vi "HUI v0.2.vi"() -> ()   [LabVIEW 2016]
uses:
  <vilib>/measure/NI_MABase.lvlib
panel:
  out "hui":dbl[](array[numeric])
  in  "wait":u32
  out "Point free":u32
  out "Point processed":u32
  in  "Quant":i32=100
  in  "stop":bool
  out "DAC FREQ/CH, Hz":dbl
  out "String":string
  in  "STOP_RUN":bool
  in  "FREQ":dbl(knob)=100.0 scale=0.0..100000.0
  in  "SIZE":dbl(knob)=1.0 scale=0.0..5.0
  # "CHANNEL A"
  # "CHANNEL B"
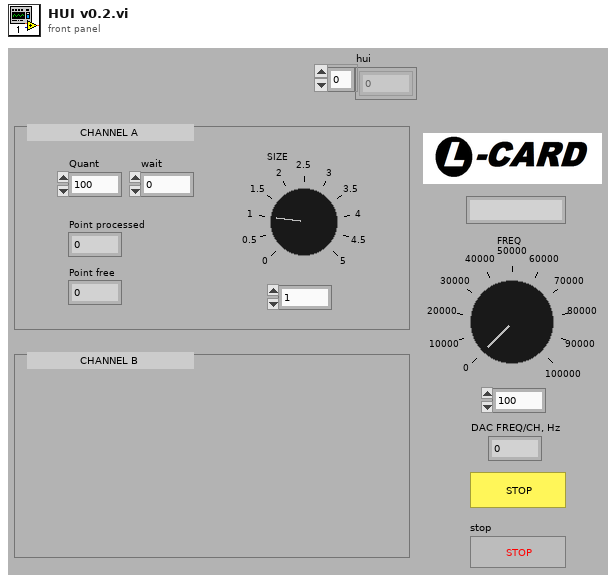
[diagram p1: front panel]
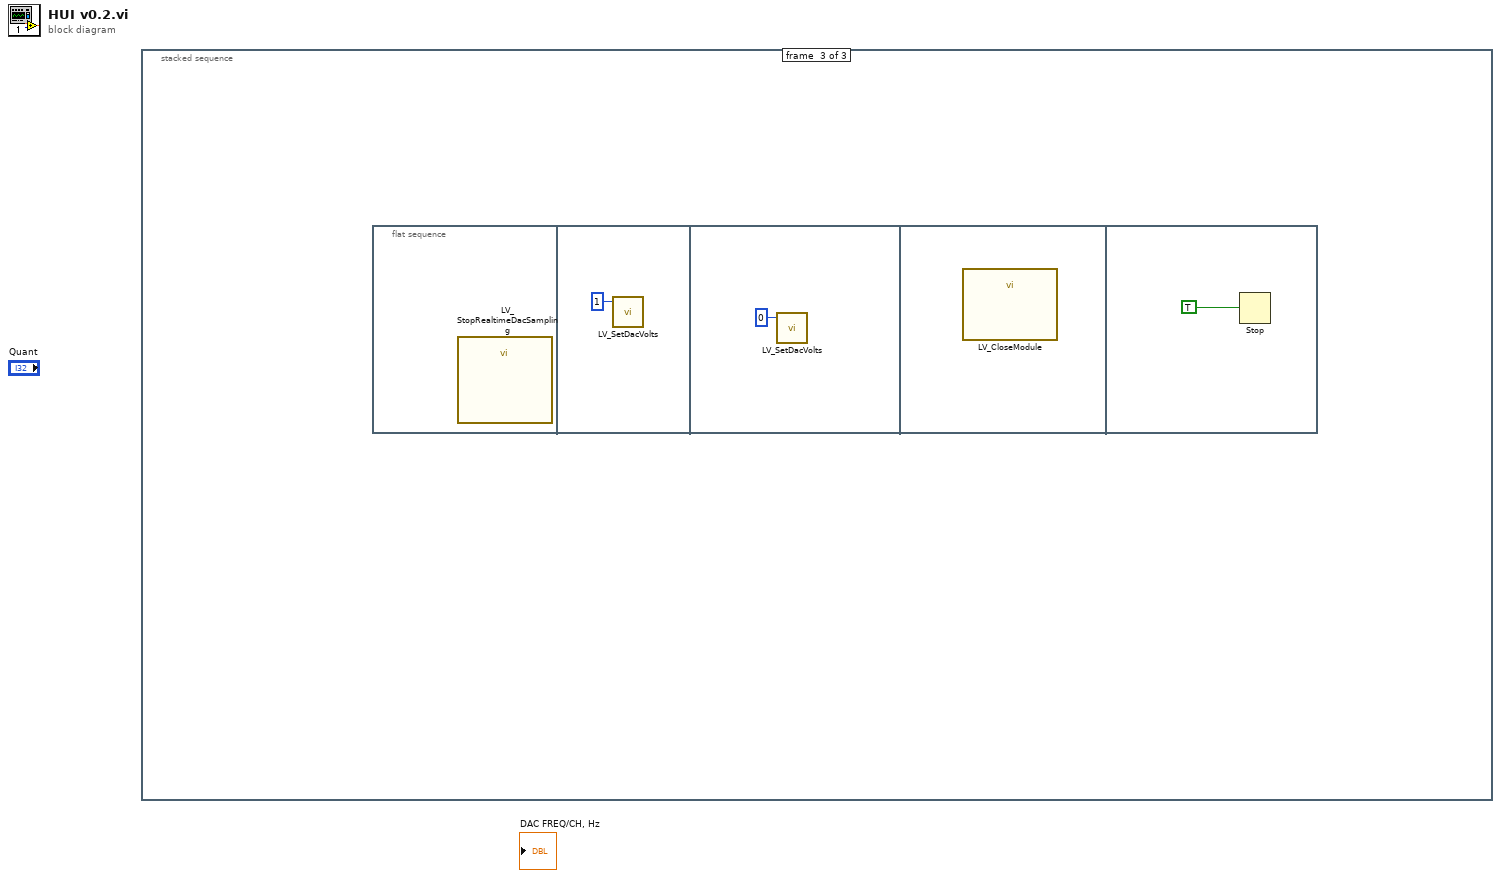
[diagram p0: block diagram]
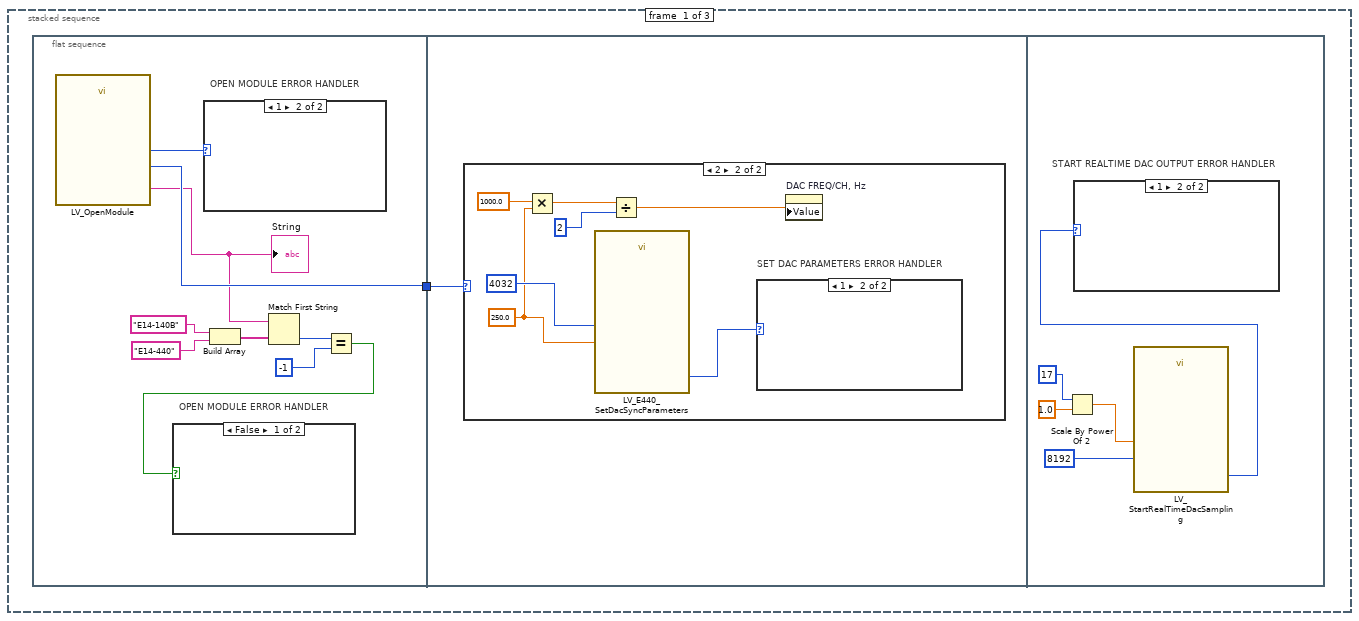
[diagram p2: hidden frame]
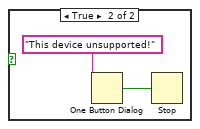
[diagram p3: hidden frame]
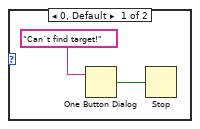
[diagram p4: hidden frame]
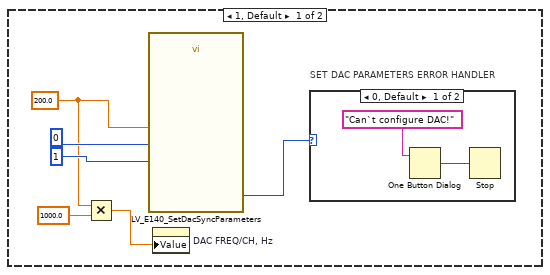
[diagram p5: hidden frame]
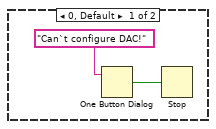
[diagram p7: hidden frame]
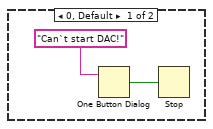
[diagram p8: hidden frame]
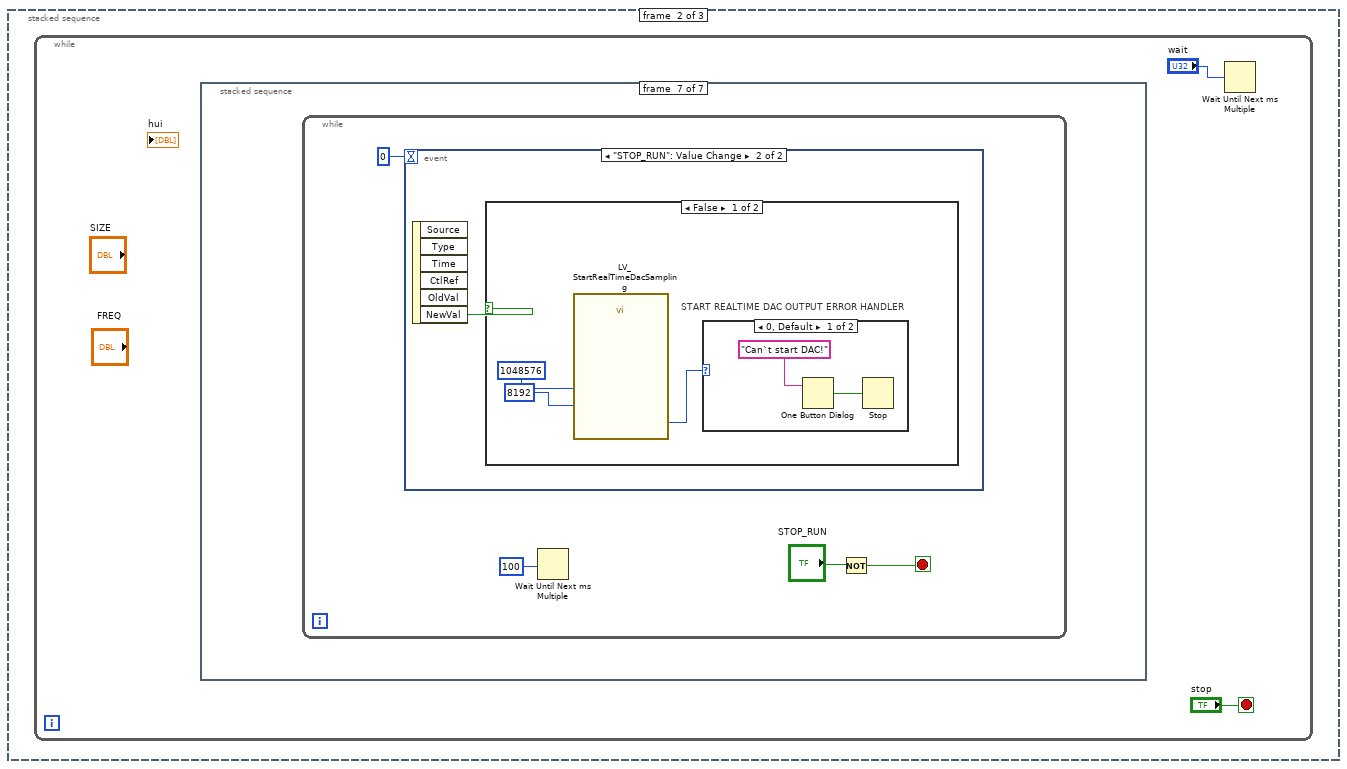
[diagram p9: hidden frame]
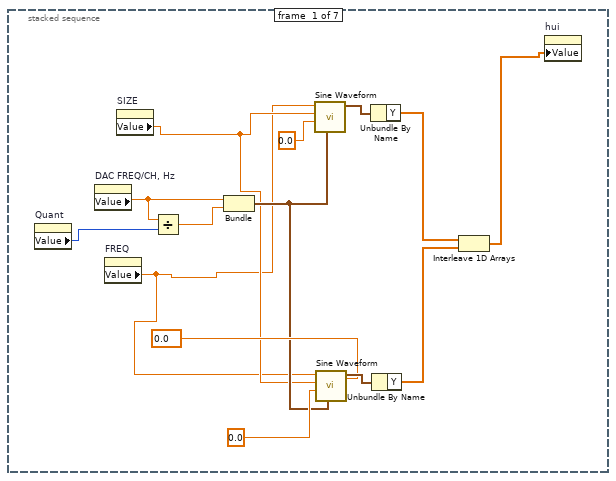
[diagram p10: hidden frame]
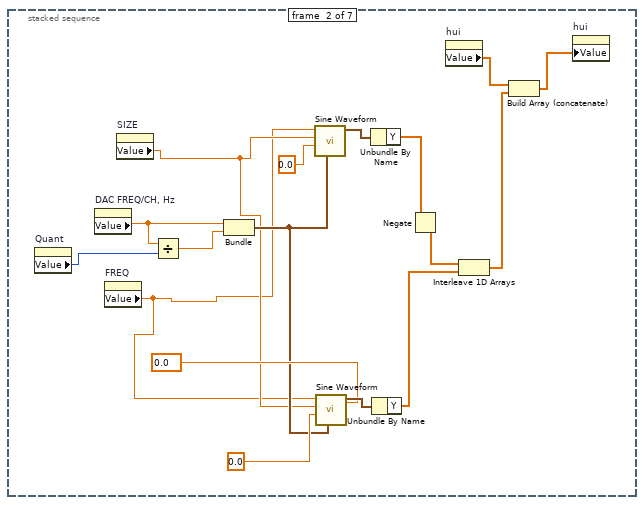
[diagram p11: hidden frame]
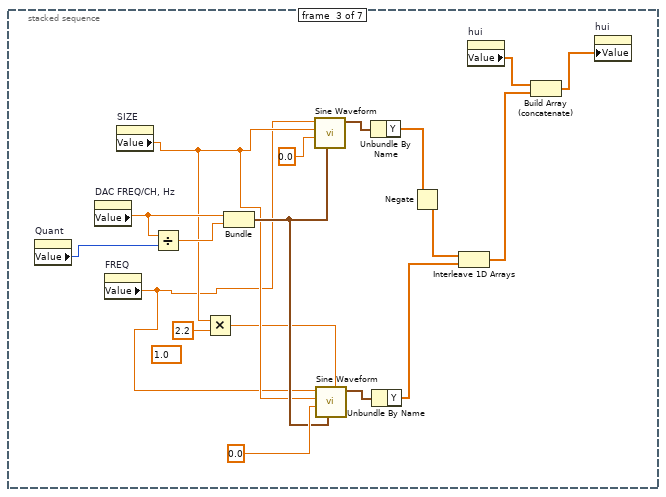
[diagram p12: hidden frame]
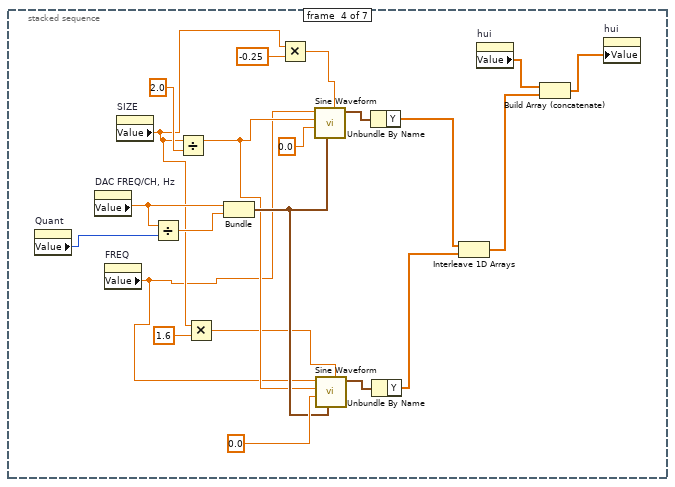
[diagram p13: hidden frame]
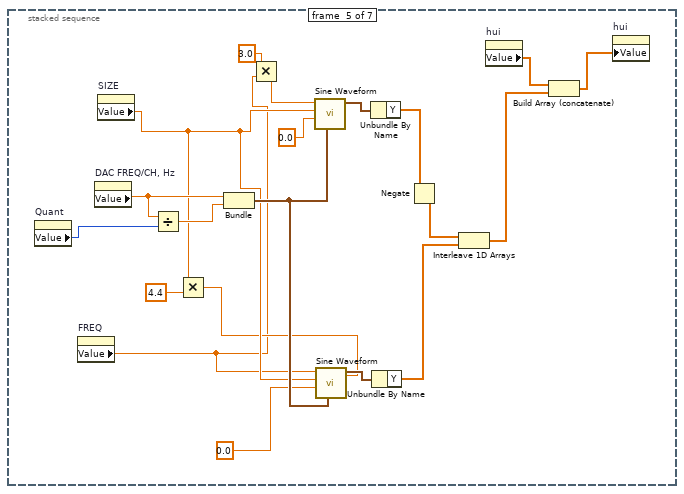
[diagram p14: hidden frame]
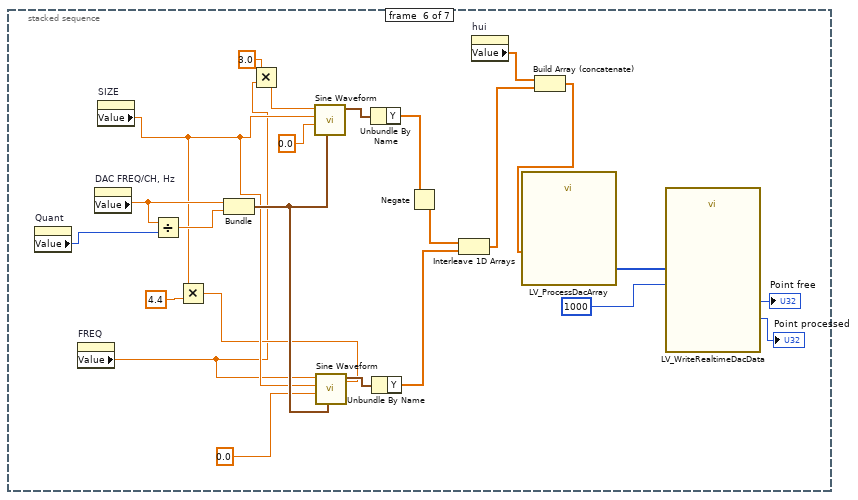
[diagram p15: hidden frame]
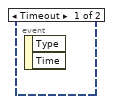
[diagram p16: hidden frame]
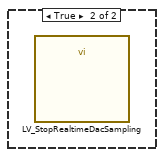
[diagram p18: hidden frame]
diagram:
  n1 = stacked-sequence {
    frame #0 {
      n2 = flat-sequence {
        tunnel: [w3] -> w1
        tunnel: w1 -> [w15]
        frame #0 {
          n3 = call <instrlib>:"LV_OpenModule.vi"() -> ("Module Name"=w2:string, "Module id"=w3:u8, "Error"=w4:u8)
          "String" <- w2
          n4 = case "OPEN MODULE ERROR HANDLER" shown="1" w4 {
            frame 0, Default {
              n5 = One Button Dialog(message="Can`t find target!") -> (true=w13:bool)  [unwired: 1 in]
              n6 = Stop(stop? (T)=w13) -> ()
            }
            frame 1 {
            }
          }
          n7 = Build Array("E14-140B", "E14-440") -> (w8:string[])
          n8 = Match First String(2:w8, 3:w2) -> (0:w7:i32)  [unwired: 1 out]
          n9 = Equal?(x=w7, y=-1) -> (x = y?=w5:bool)
          n10 = case "OPEN MODULE ERROR HANDLER" shown="False" w5 {
            frame False {
            }
            frame True {
              n11 = One Button Dialog(message="This device unsupported!") -> (true=w12:bool)  [unwired: 1 in]
              n12 = Stop(stop? (T)=w12) -> ()
            }
          }
        }
        frame #1 {
          n13 = case shown="2" w15 {
            frame 1, Default {
              w16 = 200.0
              n14 = Multiply(x=w16, y=1000.0) -> (x*y=w18:dbl)
              n15 = call <instrlib>:"LV_E140_SetDacSyncParameters.vi"("Zero on stop"=1, "Sync with ADC"=0, "Rate"=w16) -> ("Error"=w19:u32)  [unwired: 1 out]
              n16 = property on="DAC FREQ/CH, Hz" class="DigNum (strict)"("Value"=w18) -> ()  [unwired: 2 in, 2 out]
              n17 = case "SET DAC PARAMETERS ERROR HANDLER" shown="0, Default" w19 {
                frame 0, Default {
                  n18 = One Button Dialog(message="Can`t configure DAC!") -> (true=w22:bool)  [unwired: 1 in]
                  n19 = Stop(stop? (T)=w22) -> ()
                }
                frame 1 {
                }
              }
            }
            frame 2 {
              w25 = 250.0
              n20 = Multiply(x=1000.0, y=w25) -> (x*y=w26:dbl)
              n21 = call <instrlib>:"LV_E440_SetDacSyncParameters.vi"("Fifo length"=4032, "Rate"=w25) -> ("Error"=w27:u32)  [unwired: 1 out]
              n22 = Divide(x=w26, y=2) -> (x/y=w30:dbl)
              n23 = case "SET DAC PARAMETERS ERROR HANDLER" shown="1" w27 {
                frame 0, Default {
                  n24 = One Button Dialog(message="Can`t configure DAC!") -> (true=w31:bool)  [unwired: 1 in]
                  n25 = Stop(stop? (T)=w31) -> ()
                }
                frame 1 {
                }
              }
              n26 = property on="DAC FREQ/CH, Hz" class="DigNum (strict)"("Value"=w30) -> ()  [unwired: 2 in, 2 out]
            }
          }
        }
        frame #2 {
          n27 = Scale By Power Of 2(n=i16 17, x=1.0) -> (x*2^n=w33:dbl)
          n28 = call <instrlib>:"LV_StartRealTimeDacSampling.vi"("Packet size"=8192, "Buffer Size"=w33) -> ("Error"=w36:u8)
          n29 = case "START REALTIME DAC OUTPUT ERROR HANDLER" shown="1" w36 {
            frame 0, Default {
              n30 = One Button Dialog(message="Can`t start DAC!") -> (true=w38:bool)  [unwired: 1 in]
              n31 = Stop(stop? (T)=w38) -> ()
            }
            frame 1 {
            }
          }
        }
      }
    }
    frame #1 {
      n32 = while {
        stop <- "stop" stop-if-true
        n33 = stacked-sequence {
          frame #0 {
            w52 = 0.0 items=["-5V"=-5.0, "-2V"=-2.0, "-1V"=-1.0, "0V"=0.0, "1V"=1.0, "2V"=2.0, "5V"=5.0] ("DC OFFSET")
            n34 = property on="Quant" class="DigNum (strict)"() -> ("Value"=w46:i32)  [unwired: 2 in, 2 out]
            n35 = property on="DAC FREQ/CH, Hz" class="DigNum (strict)"() -> ("Value"=w49:dbl)  [unwired: 2 in, 2 out]
            n36 = property on="FREQ" class="Knob (strict)"() -> ("Value"=w43:dbl)  [unwired: 2 in, 2 out]
            n37 = property on="SIZE" class="Knob (strict)"() -> ("Value"=w44:dbl)  [unwired: 2 in, 2 out]
            n38 = Divide(x=w49, y=w46) -> (x/y=w48:dbl)
            n39 = Bundle("Value"=w49, w48) -> (w45:cluster{"Value":dbl, dbl})  [unwired: 1 in]
            n40 = call <vilib>:"Sine Waveform.vi"("sampling info"=w45, "phase"=sgl 0.0, "amplitude"=w44, "frequency"=w43) -> ("signal out"=w55:waveform(dbl))  [unwired: 6 in, 1 out]
            n41 = call <vilib>:"Sine Waveform.vi"("offset"=w52, "sampling info"=w45, "phase"=0.0, "amplitude"=w44, "frequency"=w43) -> ("signal out"=w53:waveform(dbl))  [unwired: 5 in, 1 out]
            n42 = Unbundle By Name(w55) -> ("Y"=w51:dbl[])
            n43 = Unbundle By Name(w53) -> ("Y"=w50:dbl[])
            n44 = Interleave 1D Arrays(w51, w50) -> (w42:dbl[])
            n45 = property on="hui" class="Arr (strict)"("Value"=w42) -> ()  [unwired: 2 in, 2 out]
          }
          frame #1 {
            w69 = 0.0 items=["-5V"=-5.0, "-2V"=-2.0, "-1V"=-1.0, "0V"=0.0, "1V"=1.0, "2V"=2.0, "5V"=5.0] ("DC OFFSET")
            n46 = property on="Quant" class="DigNum (strict)"() -> ("Value"=w63:i32)  [unwired: 2 in, 2 out]
            n47 = property on="DAC FREQ/CH, Hz" class="DigNum (strict)"() -> ("Value"=w66:dbl)  [unwired: 2 in, 2 out]
            n48 = property on="FREQ" class="Knob (strict)"() -> ("Value"=w60:dbl)  [unwired: 2 in, 2 out]
            n49 = property on="SIZE" class="Knob (strict)"() -> ("Value"=w61:dbl)  [unwired: 2 in, 2 out]
            n50 = Divide(x=w66, y=w63) -> (x/y=w65:dbl)
            n51 = Bundle("Value"=w66, w65) -> (w62:cluster{"Value":dbl, dbl})  [unwired: 1 in]
            n52 = call <vilib>:"Sine Waveform.vi"("sampling info"=w62, "phase"=sgl 0.0, "amplitude"=w61, "frequency"=w60) -> ("signal out"=w72:waveform(dbl))  [unwired: 6 in, 1 out]
            n53 = call <vilib>:"Sine Waveform.vi"("offset"=w69, "sampling info"=w62, "phase"=0.0, "amplitude"=w61, "frequency"=w60) -> ("signal out"=w70:waveform(dbl))  [unwired: 5 in, 1 out]
            n54 = Unbundle By Name(w72) -> ("Y"=w68:dbl[])
            n55 = Unbundle By Name(w70) -> ("Y"=w67:dbl[])
            n56 = Negate(x=w68) -> (-x=w58:dbl[])
            n57 = property on="hui" class="Arr (strict)"() -> ("Value"=w57:dbl[])  [unwired: 2 in, 2 out]
            n58 = Interleave 1D Arrays(w58, w67) -> (w59:dbl[])
            n59 = Build Array (concatenate)(w57, w59) -> (w56:dbl[])
            n60 = property on="hui" class="Arr (strict)"("Value"=w56) -> ()  [unwired: 2 in, 2 out]
          }
          frame #2 {
            (unwired) 1.0 items=["-5V"=-5.0, "-2V"=-2.0, "-1V"=-1.0, "0V"=0.0, "1V"=1.0, "2V"=2.0, "5V"=5.0] ("DC OFFSET")
            n61 = property on="Quant" class="DigNum (strict)"() -> ("Value"=w82:i32)  [unwired: 2 in, 2 out]
            n62 = property on="DAC FREQ/CH, Hz" class="DigNum (strict)"() -> ("Value"=w85:dbl)  [unwired: 2 in, 2 out]
            n63 = property on="FREQ" class="Knob (strict)"() -> ("Value"=w76:dbl)  [unwired: 2 in, 2 out]
            n64 = property on="SIZE" class="Knob (strict)"() -> ("Value"=w78:dbl)  [unwired: 2 in, 2 out]
            n65 = Divide(x=w85, y=w82) -> (x/y=w84:dbl)
            n66 = Multiply(x=w78, y=2.2) -> (x*y=w77:dbl)
            n67 = Bundle("Value"=w85, w84) -> (w81:cluster{"Value":dbl, dbl})  [unwired: 1 in]
            n68 = call <vilib>:"Sine Waveform.vi"("sampling info"=w81, "phase"=sgl 0.0, "amplitude"=w78, "frequency"=w76) -> ("signal out"=w90:waveform(dbl))  [unwired: 6 in, 1 out]
            n69 = call <vilib>:"Sine Waveform.vi"("offset"=w77, "sampling info"=w81, "phase"=0.0, "amplitude"=w78, "frequency"=w76) -> ("signal out"=w88:waveform(dbl))  [unwired: 5 in, 1 out]
            n70 = Unbundle By Name(w90) -> ("Y"=w87:dbl[])
            n71 = Unbundle By Name(w88) -> ("Y"=w86:dbl[])
            n72 = Negate(x=w87) -> (-x=w80:dbl[])
            n73 = Interleave 1D Arrays(w80, w86) -> (w73:dbl[])
            n74 = property on="hui" class="Arr (strict)"() -> ("Value"=w75:dbl[])  [unwired: 2 in, 2 out]
            n75 = Build Array (concatenate)(w75, w73) -> (w74:dbl[])
            n76 = property on="hui" class="Arr (strict)"("Value"=w74) -> ()  [unwired: 2 in, 2 out]
          }
          frame #3 {
            n77 = property on="Quant" class="DigNum (strict)"() -> ("Value"=w103:i32)  [unwired: 2 in, 2 out]
            n78 = property on="DAC FREQ/CH, Hz" class="DigNum (strict)"() -> ("Value"=w106:dbl)  [unwired: 2 in, 2 out]
            n79 = property on="FREQ" class="Knob (strict)"() -> ("Value"=w94:dbl)  [unwired: 2 in, 2 out]
            n80 = property on="SIZE" class="Knob (strict)"() -> ("Value"=w96:dbl)  [unwired: 2 in, 2 out]
            n81 = Divide(x=w106, y=w103) -> (x/y=w105:dbl)
            n82 = Divide(x=w96, y=2.0) -> (x/y=w101:dbl)
            n83 = Multiply(x=w96, y=1.6) -> (x*y=w98:dbl)
            n84 = Bundle("Value"=w106, w105) -> (w102:cluster{"Value":dbl, dbl})  [unwired: 1 in]
            n85 = Multiply(x=w96, y=-0.25) -> (x*y=w95:dbl)
            n86 = call <vilib>:"Sine Waveform.vi"("offset"=w95, "sampling info"=w102, "phase"=sgl 0.0, "amplitude"=w101, "frequency"=w94) -> ("signal out"=w111:waveform(dbl))  [unwired: 5 in, 1 out]
            n87 = call <vilib>:"Sine Waveform.vi"("offset"=w98, "sampling info"=w102, "phase"=0.0, "amplitude"=w101, "frequency"=w94) -> ("signal out"=w109:waveform(dbl))  [unwired: 5 in, 1 out]
            n88 = Unbundle By Name(w111) -> ("Y"=w108:dbl[])
            n89 = Unbundle By Name(w109) -> ("Y"=w107:dbl[])
            n90 = Interleave 1D Arrays(w108, w107) -> (w91:dbl[])
            n91 = property on="hui" class="Arr (strict)"() -> ("Value"=w92:dbl[])  [unwired: 2 in, 2 out]
            n92 = Build Array (concatenate)(w92, w91) -> (w93:dbl[])
            n93 = property on="hui" class="Arr (strict)"("Value"=w93) -> ()  [unwired: 2 in, 2 out]
          }
          frame #4 {
            n94 = property on="Quant" class="DigNum (strict)"() -> ("Value"=w124:i32)  [unwired: 2 in, 2 out]
            n95 = property on="FREQ" class="Knob (strict)"() -> ("Value"=w116:dbl)  [unwired: 2 in, 2 out]
            n96 = property on="DAC FREQ/CH, Hz" class="DigNum (strict)"() -> ("Value"=w126:dbl)  [unwired: 2 in, 2 out]
            n97 = property on="SIZE" class="Knob (strict)"() -> ("Value"=w120:dbl)  [unwired: 2 in, 2 out]
            n98 = Divide(x=w126, y=w124) -> (x/y=w125:dbl)
            n99 = Multiply(x=w120, y=4.4) -> (x*y=w119:dbl)
            n100 = Bundle("Value"=w126, w125) -> (w123:cluster{"Value":dbl, dbl})  [unwired: 1 in]
            n101 = Multiply(x=3.0 ("frequency"), y=w116) -> (x*y=w117:dbl)
            n102 = call <vilib>:"Sine Waveform.vi"("sampling info"=w123, "phase"=sgl 0.0, "amplitude"=w120, "frequency"=w117) -> ("signal out"=w131:waveform(dbl))  [unwired: 6 in, 1 out]
            n103 = call <vilib>:"Sine Waveform.vi"("offset"=w119, "sampling info"=w123, "phase"=0.0, "amplitude"=w120, "frequency"=w116) -> ("signal out"=w129:waveform(dbl))  [unwired: 5 in, 1 out]
            n104 = Unbundle By Name(w131) -> ("Y"=w128:dbl[])
            n105 = Unbundle By Name(w129) -> ("Y"=w127:dbl[])
            n106 = Negate(x=w128) -> (-x=w115:dbl[])
            n107 = Interleave 1D Arrays(w115, w127) -> (w112:dbl[])
            n108 = property on="hui" class="Arr (strict)"() -> ("Value"=w114:dbl[])  [unwired: 2 in, 2 out]
            n109 = Build Array (concatenate)(w114, w112) -> (w113:dbl[])
            n110 = property on="hui" class="Arr (strict)"("Value"=w113) -> ()  [unwired: 2 in, 2 out]
          }
          frame #5 {
            n111 = property on="Quant" class="DigNum (strict)"() -> ("Value"=w146:i32)  [unwired: 2 in, 2 out]
            n112 = property on="FREQ" class="Knob (strict)"() -> ("Value"=w138:dbl)  [unwired: 2 in, 2 out]
            n113 = property on="DAC FREQ/CH, Hz" class="DigNum (strict)"() -> ("Value"=w150:dbl)  [unwired: 2 in, 2 out]
            n114 = property on="SIZE" class="Knob (strict)"() -> ("Value"=w142:dbl)  [unwired: 2 in, 2 out]
            n115 = Divide(x=w150, y=w146) -> (x/y=w149:dbl)
            n116 = Multiply(x=w142, y=4.4) -> (x*y=w141:dbl)
            n117 = Bundle("Value"=w150, w149) -> (w145:cluster{"Value":dbl, dbl})  [unwired: 1 in]
            n118 = Multiply(x=3.0 ("frequency"), y=w138) -> (x*y=w139:dbl)
            n119 = call <vilib>:"Sine Waveform.vi"("sampling info"=w145, "phase"=sgl 0.0, "amplitude"=w142, "frequency"=w139) -> ("signal out"=w155:waveform(dbl))  [unwired: 6 in, 1 out]
            n120 = call <vilib>:"Sine Waveform.vi"("offset"=w141, "sampling info"=w145, "phase"=0.0, "amplitude"=w142, "frequency"=w138) -> ("signal out"=w153:waveform(dbl))  [unwired: 5 in, 1 out]
            n121 = Unbundle By Name(w155) -> ("Y"=w152:dbl[])
            n122 = Unbundle By Name(w153) -> ("Y"=w151:dbl[])
            n123 = Negate(x=w152) -> (-x=w137:dbl[])
            n124 = Interleave 1D Arrays(w137, w151) -> (w132:dbl[])
            n125 = property on="hui" class="Arr (strict)"() -> ("Value"=w134:dbl[])  [unwired: 2 in, 2 out]
            n126 = Build Array (concatenate)(w134, w132) -> (w133:dbl[])
            n127 = call <instrlib>:"LV_ProcessDacArray.vi"("Input data"=w133) -> ("Output data"=w148:i16[])
            n128 = call <instrlib>:"LV_WriteRealtimeDacData.vi"("Timeout"=1000, "Data"=w148) -> ("Point free"=→"Point free":u32, "Point processed"=→"Point processed":u32)  [unwired: 2 in, 1 out]
          }
          frame #6 {
            n129 = while {
              stop <- w156 stop-if-true
              n130 = event shown="[1] \"STOP_RUN\": Value Change" {
                selector: _ -> [_ _]
                dyn-events: _ -> [_ _]
                timeout: 0 -> [_ _]
                event Timeout {
                  n131 = event-data() -> ()  [unwired: 1 in, 2 out]
                }
                event "STOP_RUN": Value Change {
                  n132 = event-data() -> ("NewVal"=w160:bool)  [unwired: 1 in, 5 out]
                  n133 = case shown="False" w160 {
                    frame False {
                      n134 = call <instrlib>:"LV_StartRealTimeDacSampling.vi"("Packet size"=8192, "Buffer Size"=1048576) -> ("Error"=w161:u8)
                      n135 = case "START REALTIME DAC OUTPUT ERROR HANDLER" shown="0, Default" w161 {
                        frame 0, Default {
                          n136 = One Button Dialog(message="Can`t start DAC!") -> (true=w164:bool)  [unwired: 1 in]
                          n137 = Stop(stop? (T)=w164) -> ()
                        }
                        frame 1 {
                        }
                      }
                    }
                    frame True {
                      n138 = call <instrlib>:"LV_StopRealtimeDacSampling.vi"() -> ()  [unwired: 1 in]
                    }
                  }
                }
              }
              n139 = Wait Until Next ms Multiple(millisecond multiple=100) -> ()  [unwired: 1 out]
              n140 = Not(x="STOP_RUN") -> (.not. x?=w156:bool)
            }
          }
        }
        n141 = Wait Until Next ms Multiple(millisecond multiple="wait") -> ()  [unwired: 1 out]
      }
    }
    frame #2 {
      n142 = flat-sequence {
        frame #0 {
          n143 = call <instrlib>:"LV_StopRealtimeDacSampling.vi"() -> ()  [unwired: 1 in]
        }
        frame #1 {
          n144 = call <instrlib>:"LV_SetDacVolts.vi"("Channel Num"=u32 1) -> ()  [unwired: 2 in]
        }
        frame #2 {
          n145 = call <instrlib>:"LV_SetDacVolts.vi"("Channel Num"=u32 0) -> ()  [unwired: 2 in]
        }
        frame #3 {
          n146 = call <instrlib>:"LV_CloseModule.vi"() -> ()  [unwired: 1 in]
        }
        frame #4 {
          n147 = Stop(stop? (T)=TRUE) -> ()
        }
      }
    }
  }
